vi "Check for Single Session.vi"(7 "perform check":bool, 8 "error in":errorcluster, 11 "sessions in":variant[](array[variant])) -> (0 "error out":errorcluster, 3 "sessions out":variant[](array[variant]))   [LabVIEW 2020, in "MeasurementLink Session Management.lvlib" / "Session Reservation.lvclass"]
uses:
  Session Reservation.lvclass
  Session Reservation.lvclass/Session Reservation.ctl
  MeasurementLink Measurement Server/Helpers/Error Strings Global Internal.vi
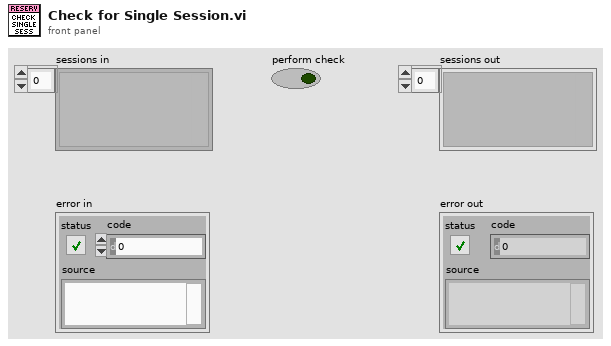
[diagram p1: front panel]
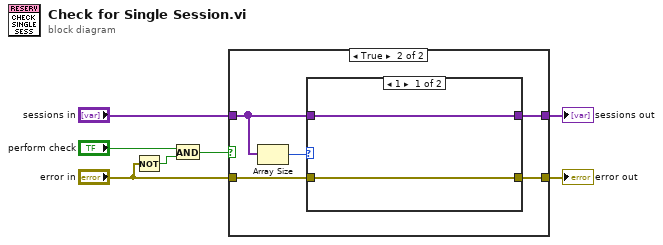
[diagram p0: block diagram]
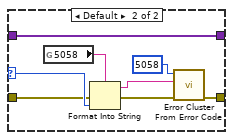
[diagram p3: hidden frame]
diagram:
  n1 = Not(x="error in") -> (.not. x?=w4:bool)
  n2 = And(x="perform check", y=w4) -> (x .and. y?=w2:bool)
  n3 = case shown="True" w2 {
    tunnel: "sessions in" -> [w9 w13]
    tunnel: [w9 w12] -> w6
    tunnel: [w8 w11] -> w5
    tunnel: "error in" -> [w8 w10]
    frame False {
    }
    frame True {
      n4 = Array Size(array=w13) -> (size(s)=w14:i32)
      n5 = case shown="1" w14 {
        selector: w14 -> [_ w22]
        tunnel: [w16 w23] -> w11
        tunnel: w13 -> [w15 w17]
        tunnel: w10 -> [w16 w20]
        tunnel: [w15 w17] -> w12
        frame 1 {
        }
        frame Default {
          n6 = global read "Error Strings Global Internal.vi" "5058"() -> (w21:string)
          n7 = Format Into String(format string=w21, error in=w20, w22) -> (resulting string=w18:string, error out=w19:errorcluster)  [unwired: 1 in]
          n8 = call <vilib>:"Error Cluster From Error Code.vi"("error in (no error)"=w19, "error message (\"\")"=w18, "error code (0)"=5058) -> ("error out"=w23:errorcluster)  [unwired: 6 in]
        }
      }
    }
  }
  "sessions out" <- w6
  "error out" <- w5
